vi "TSV path to SET.vi"(1 "*.tsv path":path) -> (0 "*.set path":path)   [LabVIEW 2023]
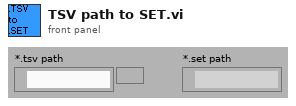
[diagram p1: front panel]
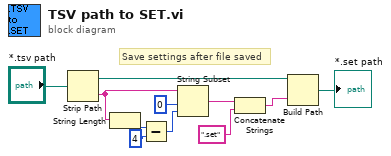
[diagram p0: block diagram]
diagram:
  # "Save settings after file saved"
  n1 = Strip Path(path="*.tsv path") -> (stripped path=w11:path, name=w6:string)
  n2 = String Length(string=w6) -> (length=w5:i32)
  n3 = Subtract(x=w5, y=4) -> (x-y=w4:i32)
  n4 = String Subset(string=w6, offset (0)=0, length (rest)=w4) -> (substring=w8:string)
  n5 = Concatenate Strings(w8, ".set") -> (w9:string)
  n6 = Build Path(base path=w11, name or relative path=w9) -> (appended path=→"*.set path":path)
